vi "Simple_REPL_Comm2.vi"(8 "REPL Name":string="Backpack", 9 "CodeRef":refnum<vi>, 11 "Microprocessor in":T1) -> (3 "Microprocessor out":T1)   [LabVIEW 2016]
uses:
  uPythonX/uPythonX.xctl
  uPythonX/PythonData.ctl
  <vilib>/event_ctls.llb/eventvkey.ctl
  <vilib>/Utility/miscctls.llb/LVPointTypeDef.ctl
panel:
  in  "Help Button":bool
  in  "Find Port":bool
  out "return?":bool
  in  "Board":bool
  out "mouse down?":bool
  in  "Port":string
  out "rows":string
  in  "View":u16(ring) items=["Complete Code"]
  in  "Spaces":bool
  in  "HelpCode":string
  in  "Code":string
  out "Script":string
  in  "Copy":bool
  out "String":string
  in  "Run":bool
  in  "Clear":bool
  in  "Run DIrect":bool
  out "FullCode":string
  out "Origin":T2
  out "Console":string
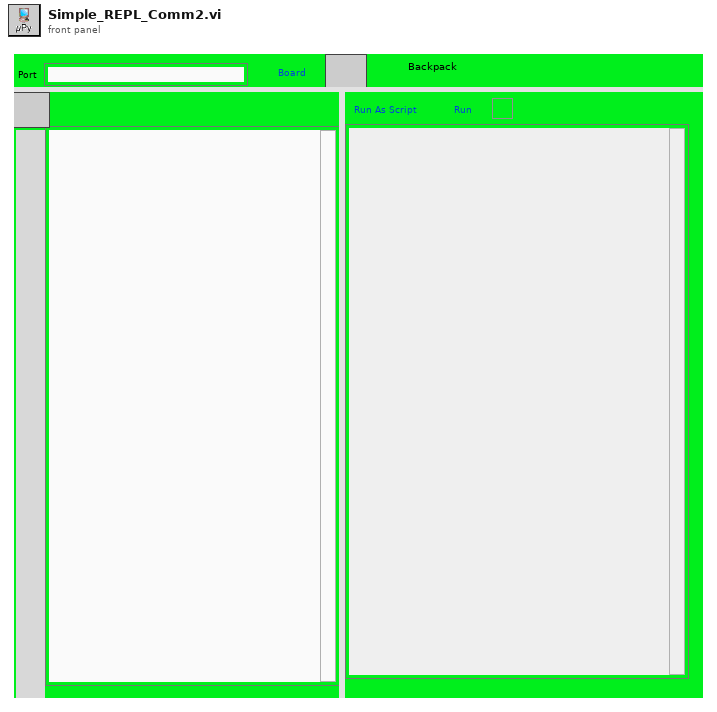
[diagram p1: front panel]
types:
  T1 = cluster{"VISA Refnum in":refnum<visa-resource-name>, "Python Code":string}
  T2 = typedef "LVPointTypeDef.ctl" = cluster{"Horizontal":i16, "Vertical":i16}
  T3 = typedef "uPythonX.xctl/PythonData.ctl" = cluster{"Port":refnum<visa-resource-name>, "All Code":string}
  T4 = typedef "eventvkey.ctl" = enum16{"ASCII", "Enter", "Return", "Shift", "Ctrl", "Alt", "Cmd", "Opt", "Caps", "NumLock", "Clear", "Break", "Up", "Down", "Left", "Right", "Insert", "Delete", "Home", "End", "PageUp", "PageDown", "Escape", "Help", "Pause", "ScrollLock", "F1", "F2", "F3", "F4", "F5", "F6", "F7", "F8", "F9", "F10", "F11", "F12", "F13", "F14", "F15", "F16", "F17", "F18", "F19", "F20", "F21", "F22", "F23", "F24", "Play", "VolumeUp", "VolumeDown", "Mute", "Two Byte Char"}
  T5 = cluster{"Shift":bool, "Ctrl":bool, "Alt":bool, "Cmd":bool, "Opt":bool}
  T6 = cluster{"Char":i16, "VKey":T4, "ScanCode":i16, "Mods":cluster{"Num Pad":bool, "Menu Key":bool}, "PlatMods":cluster{"Shift":bool, "Ctrl":bool, "Alt":bool, "Cmd":bool, "Opt":bool}, "FocusObj":refnum<vi>}
  T7 = enum16{"Left Button", "Center Button", "Right Button", "Window Close"}
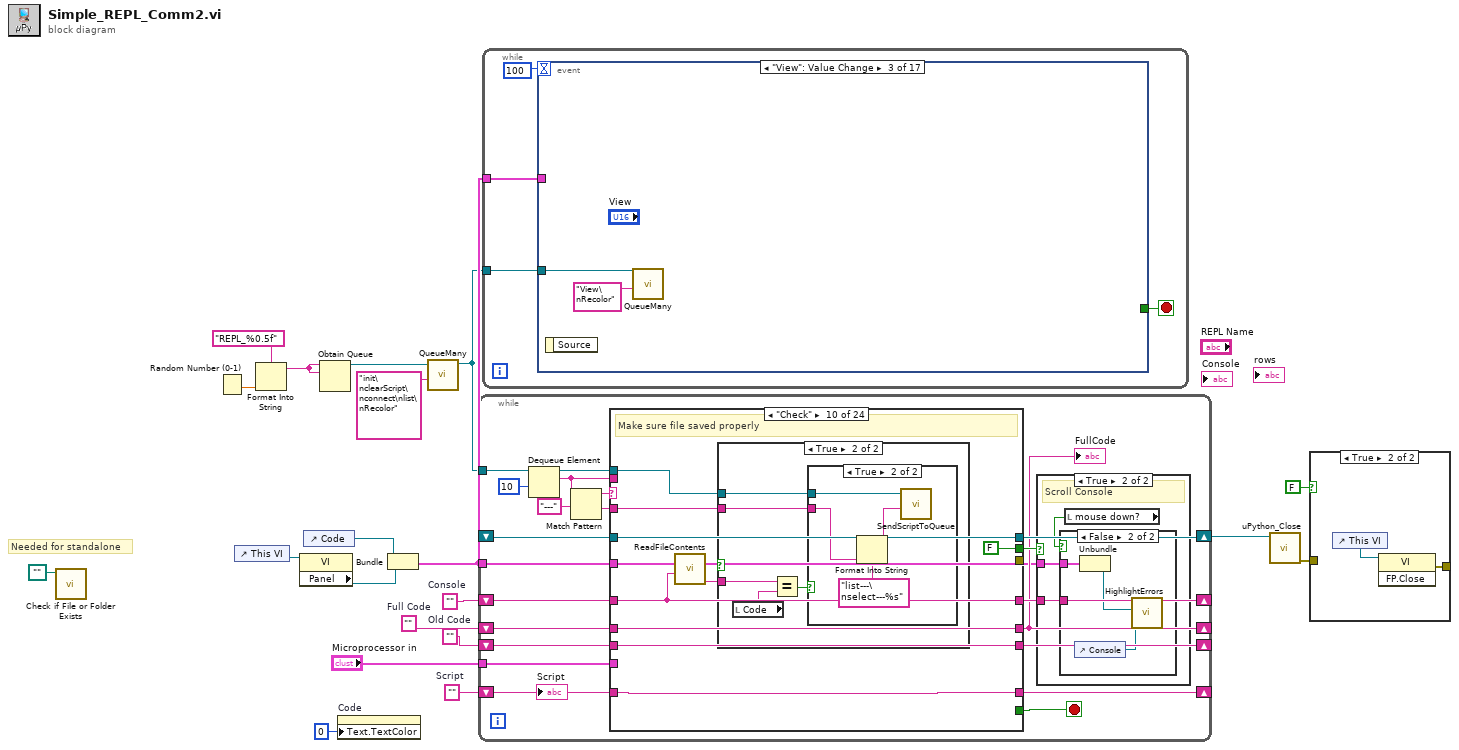
[diagram p0: block diagram]
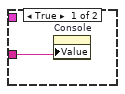
[diagram p4: hidden frame]
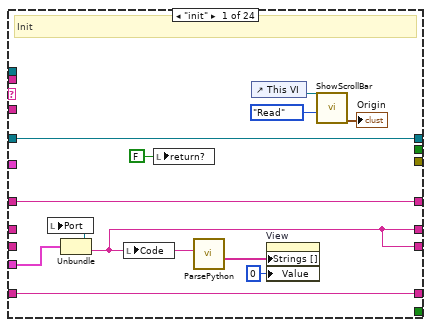
[diagram p5: hidden frame]
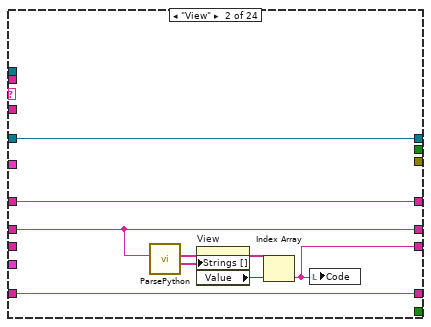
[diagram p6: hidden frame]
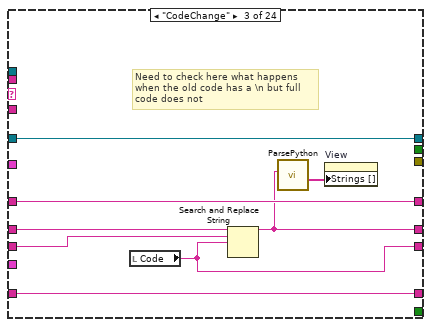
[diagram p7: hidden frame]
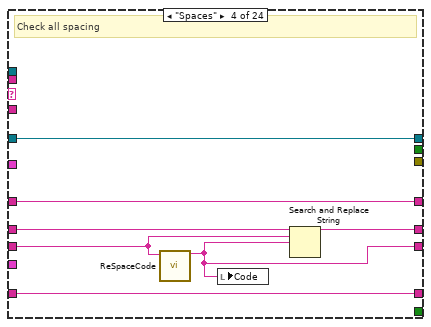
[diagram p8: hidden frame]
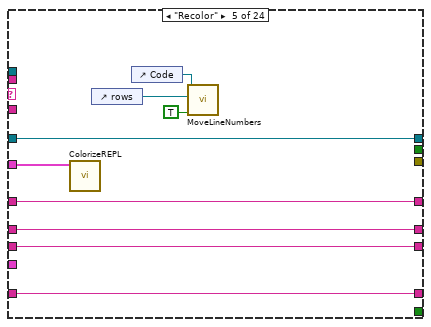
[diagram p9: hidden frame]
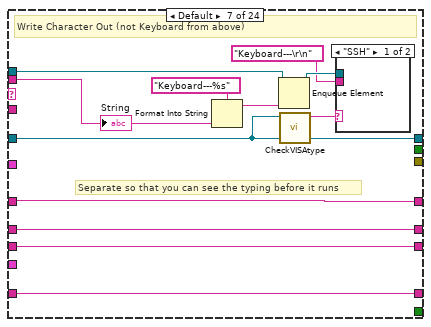
[diagram p11: hidden frame]
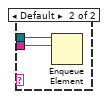
[diagram p12: hidden frame]
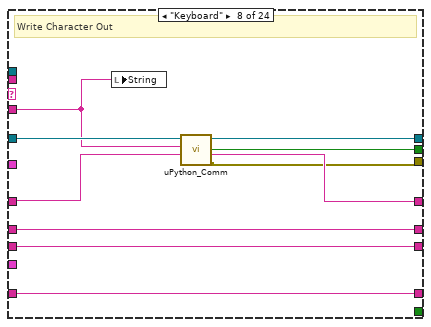
[diagram p13: hidden frame]
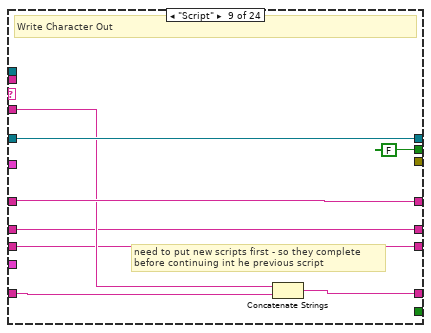
[diagram p14: hidden frame]
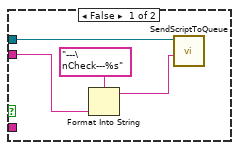
[diagram p15: hidden frame]
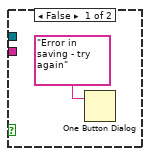
[diagram p16: hidden frame]
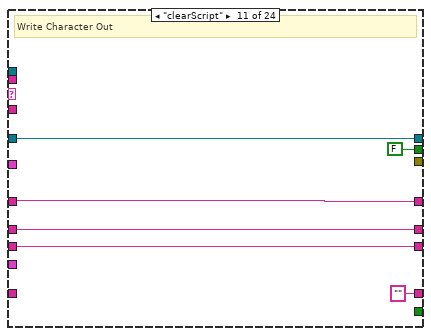
[diagram p17: hidden frame]
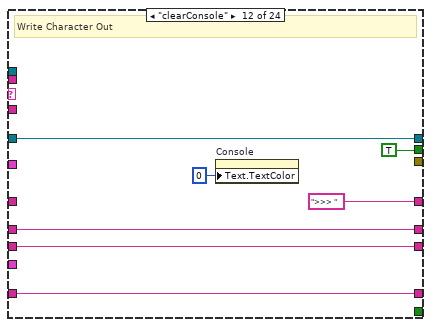
[diagram p18: hidden frame]
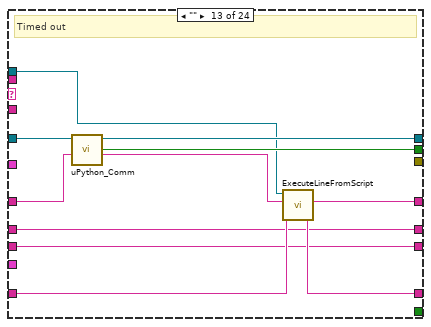
[diagram p19: hidden frame]
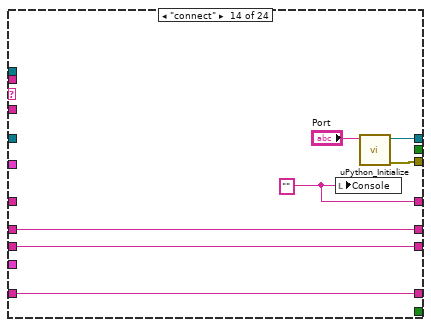
[diagram p20: hidden frame]
diagram:
  w6 = ""  # Old Code
  w7 = ""  # Full Code
  w15 = ""  # Script
  w16 = ""  # Console
  # "Needed for standalone"
  n1 = call <vilib>:"Check if File or Folder Exists.vi"("path"=path "") -> ()  [unwired: 8 in, 3 out]
  n2 = Random Number (0-1)() -> (number: 0 to 1=w10:dbl)
  n3 = control-ref of="This VI"() -> (w5:refnum<vi>)
  n4 = Format Into String(format string="REPL_%0.5f" ("name (unnamed)"), w10) -> (resulting string=w9:string)  [unwired: 2 in, 1 out]
  n5 = property class="VI"(reference=w5) -> ("Panel"=w3:refnum<vi>)  [unwired: 1 in, 2 out]
  n6 = control-ref of="Code"() -> (w4:refnum<vi>)
  n7 = Obtain Queue(name (unnamed)=w9, element data type=w9) -> (queue out=w19:refnum<queue>)  [unwired: 3 in, 2 out]
  n8 = property on="Code" class="Str"("Text.TextColor"=u32 0 ("Text.Text Colors:Text Color")) -> ()  [unwired: 2 in, 2 out]
  n9 = Bundle("Code"=w4, "Panel"=w3) -> (w20:cluster{"Code":refnum<vi>, "Panel":refnum<vi>})  [unwired: 1 in]
  n10 = call "QueueMany.vi"("Playlist"="init\nclearScript\nconnect\nlist\nRecolor" ("element"), "Queue in"=w19) -> ("Queue out"=w18:refnum<queue>)  [unwired: 9 in]
  n11 = while {
    tunnel: w18 -> [w41]
    shift-right: [w31] -> w17
    shift-left: _ -> [w39]
    shift-right: [w30] -> _
    shift-left: w16 -> [w32]
    shift-right: [w28] -> _
    shift-left: w15 -> [w27]
    tunnel: "Microprocessor in" -> [w26]
    shift-right: [w24] -> _
    shift-left: w7 -> [w25]
    shift-right: [w23] -> _
    shift-left: w6 -> [w22]
    tunnel: w20 -> [w21]
    stop <- w40 stop-if-true
    n12 = Dequeue Element(queue=w41, timeout in ms (-1)=10) -> (queue out=w37:refnum<queue>, element=w33:string)  [unwired: 1 in, 2 out]
    n13 = Match Pattern(string=w33, regular expression="---") -> (before substring=w35:string, after substring=w34:string)  [unwired: 1 in, 2 out]
    n14 = case shown="\"Check\"" w35 {
      tunnel: [_ _ _ _ _ _ _ _ _ _ _ _ _ _ _ _ _ _ _ _ _ _ _ TRUE] -> w40
      tunnel: w39 -> [w61 w69 w77 w84 w93 w98 w100 w121 w130 w140 w160 w167 w175 _ w186 w200 w208 w212 w240 w253 w264 w270 w276 w289]
      tunnel: w37 -> [_ _ _ _ _ _ w103 _ _ w136 _ _ w168 _ w190 w197 _ _ _ _ _ _ _ _]
      tunnel: w34 -> [_ _ _ _ _ _ _ w116 w125 w133 _ _ _ _ _ _ _ _ _ _ _ _ _ _]
      tunnel: w33 -> [_ _ _ _ _ _ w105 _ _ _ _ _ _ _ _ _ _ _ _ _ _ _ _ _]
      tunnel: [w61 w69 w77 w84 w93 w98 w100 w119 w130 w140 w160 w167 w172 w184 w186 w200 w208 w220 w244 w250 w264 w270 w276 w289] -> w31
      tunnel: w32 -> [w60 w68 w76 w83 w92 w97 w109 w120 w129 w135 w159 _ w174 _ w189 w199 w207 w215 w241 w254 w266 w272 w278 w290]
      tunnel: [w60 w68 w76 w83 w92 w97 w109 w118 w129 w135 w159 ">>> " ("Console") w173 w182 w189 w199 w207 w218 w228 w248 w266 w272 w278 w290] -> w30
      tunnel: [_ _ _ _ _ _ _ w113 _ _ _ _ _ w183 _ _ _ w217 w243 w249 _ _ _ _] -> _
      tunnel: [_ _ _ _ _ _ _ w117 FALSE ("Update?") FALSE ("Update?") FALSE ("Update?") TRUE ("Update?") w171 _ TRUE ("Update?") _ _ TRUE ("Update?") TRUE ("Update?") TRUE ("Update?") _ _ _ _] -> w29
      tunnel: [w59 w67 w75 w82 w90 w96 w110 w122 w127 w138 "" ("Script") w165 w177 w181 w191 w201 w204 w226 w246 w256 w265 w271 w277 w287] -> w28
      tunnel: w27 -> [w59 w67 w75 w82 w90 w96 w110 w122 w126 w138 _ w165 w176 w181 w191 w201 w204 w226 w246 w256 w265 w271 w277 w287]
      tunnel: w26 -> [w58 _ _ _ _ _ _ _ _ _ _ _ _ _ _ _ _ _ _ _ _ _ _ w286]
      tunnel: [w51 w65 w70 w78 w89 w95 w102 w115 w124 w132 w156 w163 w170 w180 w188 w196 w206 w211 w239 w252 w258 w268 w275 w282] -> w24
      tunnel: w25 -> [_ w65 w74 w81 w89 w95 w102 w115 w124 w132 w156 w163 w170 w180 w188 _ w206 w211 w239 w252 w258 w268 w275 w282]
      tunnel: [w51 w62 w72 w79 w91 w94 w101 w114 w123 w131 w155 w162 w169 w179 w187 w196 w205 w210 w238 w251 w257 w267 w274 w281] -> w23
      tunnel: w22 -> [_ _ w73 w80 w91 w94 w101 w114 w123 w131 w155 w162 w169 w179 w187 _ w205 w210 w238 w251 w257 w267 w274 w281]
      tunnel: w21 -> [_ _ _ _ w88 _ _ _ _ _ _ _ _ _ _ _ _ _ _ _ _ _ _ _]
      frame "init" {
        # "Init"
        n15 = Unbundle(w58) -> ("VISA Refnum in"=w54:refnum<visa-resource-name>, "Python Code"=w51:string)
        n16 = local write "Port"(w54) -> ()
        n17 = local write "Code"(w51) -> ()
        n18 = local write "return?"(FALSE ("return?")) -> ()
        n19 = call "ParsePython.vi"("String"=w51) -> ("functions"=w53:string[])  [unwired: 8 in, 2 out]
        n20 = control-ref of="This VI"() -> (w57:refnum<vi>)
        n21 = property on="View" class="Ring (strict)"("Strings []"=w53, "Value"=0 ("timeout in ms (-1)")) -> ()  [unwired: 2 in, 2 out]
        n22 = call "ShowScrollBar.vi"("Task"=enum16{"Read", "Open", "Close", "Reset"}."Read", "VI in"=w57) -> ("Origin"=→"Origin":T2)  [unwired: 9 in]
      }
      frame "View" {
        n23 = call "ParsePython.vi"("String"=w65) -> ("functions"=w64:string[], "Subs"=w63:string[])  [unwired: 8 in, 1 out]
        n24 = property on="View" class="Ring (strict)"("Strings []"=w64) -> ("Value"=w66:u16)  [unwired: 2 in, 2 out]
        n25 = Index Array(array=w63, index=w66) -> (element=w62:string)
        n26 = local write "Code"(w62) -> ()
      }
      frame "CodeChange" {
        # "Need to check here what happens\nwhen the old code has a \\n but full\ncode does not"
        n27 = local read "Code"() -> (w72:string)
        n28 = Search and Replace String(input string=w74, search string=w73, replace string=w72) -> (result string=w70:string)  [unwired: 5 in, 3 out]
        n29 = call "ParsePython.vi"("String"=w70) -> ("functions"=w71:string[])  [unwired: 8 in, 2 out]
        n30 = property on="View" class="Ring (strict)"("Strings []"=w71) -> ()  [unwired: 2 in, 2 out]
      }
      frame "Spaces" {
        # "Check all spacing"
        n31 = call "ReSpaceCode.vi"("Code"=w80) -> ("String"=w79:string)  [unwired: 10 in]
        n32 = local write "Code"(w79) -> ()
        n33 = Search and Replace String(input string=w81, search string=w80, replace string=w79) -> (result string=w78:string)  [unwired: 5 in, 3 out]
      }
      frame "Recolor" {
        n34 = call "ColorizeREPL.vi"("refs"=w88) -> ()  [unwired: 9 in, 1 out]
        n35 = control-ref of="rows"() -> (w86:refnum<vi>)
        n36 = control-ref of="Code"() -> (w87:refnum<vi>)
        n37 = call "MoveLineNumbers.vi"("Force?"=TRUE, "rows"=w86, "Code"=w87) -> ()  [unwired: 9 in]
      }
      frame "scroll" {
        # "reset row numbers"
      }
      frame Default {
        # "Separate so that you can see the typing before it runs"
        # "Write Character Out (not Keyboard from above)"
        n38 = Format Into String(format string="Keyboard---%s", w105) -> (resulting string=w107:string)  [unwired: 2 in, 1 out]
        n39 = Enqueue Element(queue=w103, element=w107) -> (queue out=w106:refnum<queue>)  [unwired: 2 in, 2 out]
        n40 = call "CheckVISAtype.vi"("VISA Refnum in"=w100) -> ("data string"=w99:string)  [unwired: 8 in, 2 out]
        n41 = case shown="\"SSH\"" w99 {
          tunnel: w106 -> [_ w112]
          tunnel: "Keyboard---\r\n" ("regular expression") -> [_ w111]
          frame "SSH" {
          }
          frame Default {
            n42 = Enqueue Element(queue=w112, element=w111) -> ()  [unwired: 2 in, 3 out]
          }
        }
        "String" <- w105
      }
      frame "Keyboard" {
        # "Write Character Out"
        n43 = local write "String"(w116) -> ()
        n44 = call "uPython_Comm.vi"("Console In"=w120, "Script"=w116, "VISA Refnum in"=w121) -> ("error out"=w113:errorcluster, "Console Out"=w118:string, "VISA out"=w119:refnum<visa-resource-name>, "Update?"=w117:bool)  [unwired: 4 in, 1 out]
      }
      frame "Script" {
        # "need to put new scripts first - so they complete\nbefore continuing int he previous script"
        # "Write Character Out"
        n45 = Concatenate Strings(w125, w126) -> (w127:string)
      }
      frame "Check" {
        # "Make sure file saved properly"
        n46 = call "ReadFileContents.vi"("Console"=w135) -> ("File Contents"=w134:string, "Success?"=w137:bool)  [unwired: 9 in]
        n47 = case shown="True" w137 {
          tunnel: w136 -> [w144 w145]
          tunnel: w134 -> [_ w148]
          tunnel: w133 -> [w142 w147]
          frame False {
            n48 = Format Into String(format string="---\nCheck---%s" ("String"), w142) -> (resulting string=w141:string)  [unwired: 2 in, 1 out]
            n49 = call "SendScriptToQueue.vi"("String"=w141, "Queue in"=w144) -> ()  [unwired: 10 in]
          }
          frame True {
            n50 = local read "Code"() -> (w149:string)
            n51 = Equal?(x=w148, y=w149) -> (x = y?=w146:bool)
            n52 = case shown="True" w146 {
              tunnel: w147 -> [_ w153]
              tunnel: w145 -> [_ w152]
              frame False {
                n53 = One Button Dialog(message="Error in saving - try again" ("Code")) -> ()  [unwired: 1 in, 1 out]
              }
              frame True {
                n54 = Format Into String(format string="list---\nselect---%s" ("element"), w153) -> (resulting string=w151:string)  [unwired: 2 in, 1 out]
                n55 = call "SendScriptToQueue.vi"("String"=w151, "Queue in"=w152) -> ()  [unwired: 10 in]
              }
            }
          }
        }
      }
      frame "clearScript" {
        # "Write Character Out"
      }
      frame "clearConsole" {
        # "Write Character Out"
        n56 = property on="Console" class="Str"("Text.TextColor"=u32 0 ("Text.Text Colors:Text Color")) -> ()  [unwired: 2 in, 2 out]
      }
      frame "" {
        # "Timed out"
        n57 = call "uPython_Comm.vi"("Console In"=w174, "VISA Refnum in"=w175) -> ("Console Out"=w173:string, "VISA out"=w172:refnum<visa-resource-name>, "Update?"=w171:bool)  [unwired: 5 in, 2 out]
        n58 = call "ExecuteLineFromScript.vi"("Script in"=w176, "Console"=w173, "Queue in"=w168) -> ("Script out"=w177:string)  [unwired: 8 in]
      }
      frame "connect" {
        w182 = "" ("element")
        n59 = local write "Console"(w182) -> ()
        n60 = call "uPython_Initialize.vi"("VISA Refnum in"="Port") -> ("error out"=w183:errorcluster, "VISA Refnum out"=w184:refnum<visa-resource-name>)  [unwired: 9 in]
      }
      frame "list" {
        # "get file listing"
        n61 = call "CheckVISAtype.vi"("VISA Refnum in"=w186) -> ("data string"=w185:string)  [unwired: 8 in, 2 out]
        n62 = case shown="Default" w185 {
          tunnel: w190 -> [w194 _]
          frame Default {
            n63 = call "SendScriptToQueue.vi"("String"="import os\nos.listdir()\n\nlisting---" ("element"), "Queue in"=w194) -> ()  [unwired: 10 in]
          }
          frame "" {
          }
        }
      }
      frame "read" {
        n64 = call "ReadFileContents.vi"("Console"=w199) -> ("File Contents"=w196:string, "Success?"=w198:bool)  [unwired: 9 in]
        n65 = local write "Code"(w196) -> ()
        n66 = case shown="False" w198 {
          tunnel: w197 -> [w203 _]
          frame False {
            n67 = call "SendScriptToQueue.vi"("String"="---\nread---", "Queue in"=w203) -> ()  [unwired: 10 in]
          }
          frame True {
          }
        }
        n68 = property on="View" class="Ring (strict)"("Val(Sgnl)"=0 ("timeout in ms (-1)")) -> ()  [unwired: 2 in, 2 out]
      }
      frame "ListDialog" {
        n69 = call "ReadFilesOnMP.vi"("VISA"=w208) -> ()  [unwired: 11 in]
      }
      frame "run" {
        w216 = "\u0003"  # Ctrl C
        w223 = "\u0004"  # Ctrl D
        # "run on main.py"
        n70 = call "uPython_Comm.vi"("Console In"=w215, "Script"=w216, "VISA Refnum in"=w212) -> ("error out"=w214:errorcluster, "VISA out"=w213:refnum<visa-resource-name>)  [unwired: 4 in, 3 out]
        n71 = local read "Code"() -> (w219:string)
        n72 = call "SavePyFile.vi"("Name"="main.py", "error in"=w214, "Python Code"=w219, "VISA in"=w213) -> ("error out"=w224:errorcluster, "Reply"=w222:string, "VISA out"=w225:refnum<visa-resource-name>)  [unwired: 5 in]
        n73 = call "uPython_Comm.vi"("error in (no error)"=w224, "Console In"=w222, "Script"=w223, "VISA Refnum in"=w225) -> ("error out"=w217:errorcluster, "Console Out"=w218:string, "VISA out"=w220:refnum<visa-resource-name>)  [unwired: 3 in, 2 out]
      }
      frame "runRaw" {
        w242 = "\u0003\u0003\u0001"  # Ctrl C,C,A
        w245 = "\u0004"  # Ctrl D
        # "run on main.py"
        n74 = call "uPython_Comm.vi"("Console In"=w241, "Script"=w242, "VISA Refnum in"=w240) -> ("error out"=w236:errorcluster, "Console Out"=w232:string, "VISA out"=w237:refnum<visa-resource-name>)  [unwired: 4 in, 2 out]
        n75 = local read "Code"() -> (w233:string)
        n76 = call "uPython_Comm.vi"("error in (no error)"=w236, "Console In"=w232, "Script"=w233, "VISA Refnum in"=w237) -> ("error out"=w235:errorcluster, "Console Out"=w231:string, "VISA out"=w234:refnum<visa-resource-name>)  [unwired: 3 in, 2 out]
        n77 = call "uPython_Comm.vi"("error in (no error)"=w235, "Console In"=w231, "Script"=w245, "VISA Refnum in"=w234) -> ("error out"=w243:errorcluster, "Console Out"=w229:string, "VISA out"=w244:refnum<visa-resource-name>)  [unwired: 3 in, 2 out]
        n78 = Concatenate Strings(w229, "\r\n" ("Script")) -> (w228:string)
      }
      frame "leaveRaw" {
        w255 = "\r\u0002"  # \r Ctrl B
        # "run on main.py"
        n79 = call "uPython_Comm.vi"("Console In"=w254, "Script"=w255, "VISA Refnum in"=w253) -> ("error out"=w249:errorcluster, "Console Out"=w248:string, "VISA out"=w250:refnum<visa-resource-name>)  [unwired: 4 in, 2 out]
      }
      frame "help" {
        n80 = local read "Code"() -> (w259:string)
        n81 = Bundle(cluster=T3 {"Port"="", "All Code"="Hi"} ("Data In"), "Port"=w264, "All Code"=w259) -> (w263:T3)
        n82 = control-ref of="HelpCode"() -> (w261:refnum<vi>)
        n83 = call "OpenHelp.vi"("Code Ref"=w261, "Data In"=w263, "Dialog"=enum16{"REPL", "Help"}."Help") -> ()  [unwired: 9 in]
      }
      frame "update" {
        n84 = property class="Str"(reference="CodeRef", "Val(Sgnl)"=w268) -> ()  [unwired: 1 in, 2 out]
      }
      frame "findPort" {
        n85 = call "GatheringSerialPortNames.vi"() -> ("name"=w273:string)  [unwired: 11 in]
        n86 = property on="Port" class="Str"("Val(Sgnl)"=w273) -> ()  [unwired: 2 in, 2 out]
      }
      frame "done" {
        n87 = property on="Code" class="Str"("Value"="" ("Code"), "Text.TextColor"=u32 0 ("Text.Text Colors:Text Color")) -> ()  [unwired: 2 in, 2 out]
        n88 = Bundle(cluster=w286, "VISA Refnum in"=w289, "Python Code"=w282) -> (→"Microprocessor out":T1)
        n89 = control-ref of="This VI"() -> (w284:refnum<vi>)
        n90 = local read "Origin"() -> (w285:T2)
        n91 = call "ShowScrollBar.vi"("Origin in"=w285, "Task"=enum16{"Read", "Open", "Close", "Reset"}."Reset", "VI in"=w284) -> ()  [unwired: 8 in, 1 out]
      }
    }
    "FullCode" <- w24
    n92 = case shown="True" w29 {
      tunnel: w30 -> [_ w44]
      tunnel: w21 -> [_ w42]
      frame False {
      }
      frame True {
        # "Scroll Console"
        n93 = local read "mouse down?"() -> (w43:bool)
        n94 = case shown="False" w43 {
          tunnel: w44 -> [w45 w49]
          tunnel: w42 -> [_ w47]
          frame True {
            n95 = property on="Console" class="Str"("Value"=w45) -> ()  [unwired: 2 in, 2 out]
          }
          frame False {
            n96 = control-ref of="Console"() -> (w48:refnum<vi>)
            n97 = Unbundle(w47) -> ("Panel"=w46:refnum<vi>)  [unwired: 1 out]
            n98 = call "HighlightErrors.vi"("String"=w49, "Front Panel"=w46, "Console"=w48) -> ()  [unwired: 9 in]
          }
        }
      }
    }
    "Script" <- w27
  }
  n99 = while {
    tunnel: w18 -> [w295]
    tunnel: w20 -> [w292]
    stop <- w294 stop-if-true
    n100 = event shown="[2] \"View\": Value Change" {
      selector: _ -> [_ _ _ _ _ _ _ _ _ _ _ _ _ _ _ _ _]
      dyn-events: _ -> [_ _ _ _ _ _ _ _ _ _ _ _ _ _ _ _ _]
      timeout: 100 -> [_ _ _ _ _ _ _ _ _ _ _ _ _ _ _ _ _]
      tunnel: w295 -> [_ w301 w304 w306 w312 w330 _ _ w340 w353 w355 w357 w358 w360 w362 _ w365]
      tunnel: [_ _ _ _ _ _ _ _ w333 _ _ _ _ _ _ _ _] -> w294
      tunnel: w292 -> [_ w300 _ _ _ _ _ _ _ _ _ _ _ _ _ _ _]
      event Timeout {
        n101 = event-data() -> ()  [unwired: 1 in, 3 out]
        n102 = control-ref of="Code"() -> (w297:refnum<vi>)
        n103 = control-ref of="rows"() -> (w298:refnum<vi>)
        n104 = call "MoveLineNumbers.vi"("Force?"=TRUE, "rows"=w298, "Code"=w297) -> ()  [unwired: 9 in]
      }
      event "Code": Value Change {
        # "Need to have these here or you can get screwy stuff happening"
        n105 = event-data() -> ()  [unwired: 1 in, 2 out]
        n106 = local read "return?"() -> (w299:bool)
        n107 = call "ColorizeREPL.vi"("refs"=w300, "Add Spaces?"=w299) -> ()  [unwired: 8 in, 1 out]
        n108 = call "QueueMany.vi"("Playlist"="CodeChange" ("element"), "Queue in"=w301) -> ()  [unwired: 9 in, 1 out]
      }
      event "View": Value Change {
        n109 = event-data() -> ()  [unwired: 1 in, 1 out]
        n110 = call "QueueMany.vi"("Playlist"="View\nRecolor" ("element"), "Queue in"=w304) -> ()  [unwired: 9 in, 1 out]
      }
      event "Spaces": Value Change {
        n111 = event-data() -> ()  [unwired: 1 in, 1 out]
        n112 = call "QueueMany.vi"("Playlist"="Spaces\nRecolor" ("element"), "Queue in"=w306) -> ()  [unwired: 9 in, 1 out]
      }
      event Key Down {
        n113 = event-data() -> ("Char"=w316:i16, "VKey"=w307:T4, "ScanCode"=w315:i16, "Mods"=w314:cluster{"Num Pad":bool, "Menu Key":bool}, "PlatMods"=w313:T5, "FocusObj"=w309:refnum<vi>)  [unwired: 1 in]
        n114 = Bundle("Char"=w316, "VKey"=w307, "ScanCode"=w315, "Mods"=w314, "PlatMods"=w313, "FocusObj"=w309) -> (w317:T6)  [unwired: 1 in]
        n115 = control-ref of="Code"() -> (w310:refnum<vi>)
        n116 = Not Equal?(x=w310, y=w309) -> (x != y?=w311:bool)
        n117 = case shown="False" w311 {
          tunnel: w317 -> [_ w324]
          tunnel: w312 -> [_ w322]
          tunnel: w307 -> [w319 _]
          tunnel: [w318 _] -> w308
          frame False {
            n118 = Equal?(x=eventvkey."Return" ("VKey"), y=w319) -> (x = y?=w318:bool)
          }
          frame True {
            n119 = call "TranslateTyping.vi"("Cluster"=w324) -> ("Script?"=w321:bool, "string"=w323:string)  [unwired: 8 in, 1 out]
            n120 = case shown="True" w321 {
              tunnel: w323 -> [w325 w328]
              tunnel: w322 -> [w326 w327]
              frame False {
                n121 = call "QueueMany.vi"("Playlist"=w325, "Queue in"=w326) -> ()  [unwired: 9 in, 1 out]
              }
              frame True {
                n122 = call "SendScriptToQueue.vi"("String"=w328, "Queue in"=w327) -> ()  [unwired: 10 in]
              }
            }
          }
        }
        "return?" <- w308
      }
      event "Copy": Value Change {
        n123 = event-data() -> ()  [unwired: 1 in, 1 out]
        n124 = call "QueueMany.vi"("Playlist"="update" ("element"), "Queue in"=w330) -> ()  [unwired: 9 in, 1 out]
      }
      event Mouse Down {
        n125 = event-data() -> ()  [unwired: 1 in, 8 out]
        "mouse down?" <- TRUE ("mouse down?")
      }
      event Mouse Leave; Mouse Up {
        n126 = event-data() -> ()  [unwired: 1 in, 4 out]
        n127 = local write "mouse down?"(FALSE ("mouse down?")) -> ()
      }
      event Panel Close? {
        n128 = event-data() -> ()  [unwired: 1 in, 1 out]
        n129 = local read "Microprocessor in"() -> (w337:T1)
        n130 = local read "Code"() -> (w336:string)
        n131 = Unbundle By Name(w337) -> ("Python Code"=w335:string)
        n132 = Not Equal?(x=w335, y=w336) -> (x != y?=w334:bool)
        n133 = case shown="True" w334 {
          tunnel: ["done" ("element") w345] -> w338
          tunnel: [TRUE ("Discard?") w344] -> w333
          frame False {
          }
          frame True {
            n134 = call "CloseDialog.vi"() -> ("Which Button?"=w343:T7)  [unwired: 11 in]
            n135 = case shown="\"Center Button\"" w343 {
              tunnel: ["update\ndone" ("element") "done" ("element") "" ("element")] -> w345
              tunnel: [TRUE ("Discard?") TRUE ("Discard?") FALSE ("Discard?")] -> w344
              frame "Left Button" {
              }
              frame "Center Button" {
              }
              frame Default {
              }
            }
          }
        }
        n136 = call "QueueMany.vi"("Playlist"=w338, "Queue in"=w340) -> ()  [unwired: 9 in, 1 out]
        n137 = event-data("Discard?"=TRUE) -> ()  [unwired: 1 in, 1 out]
      }
      event "Board": Value Change {
        n138 = event-data() -> ()  [unwired: 1 in, 1 out]
        n139 = call "QueueMany.vi"("Playlist"="ListDialog" ("element"), "Queue in"=w353) -> ()  [unwired: 9 in, 1 out]
      }
      event "Find Port": Value Change {
        n140 = event-data() -> ()  [unwired: 1 in, 1 out]
        n141 = call "QueueMany.vi"("Playlist"="findPort" ("element"), "Queue in"=w355) -> ()  [unwired: 9 in, 1 out]
      }
      event "Run DIrect": Value Change {
        n142 = event-data() -> ()  [unwired: 1 in, 1 out]
        n143 = call "SendScriptToQueue.vi"("String"="Code", "Queue in"=w357) -> ()  [unwired: 10 in]
      }
      event "Run": Value Change {
        n144 = event-data() -> ()  [unwired: 1 in, 1 out]
        n145 = call "QueueMany.vi"("Playlist"="runRaw" ("element"), "Queue in"=w358) -> ()  [unwired: 9 in, 1 out]
      }
      event "Port": Value Change {
        n146 = event-data() -> ()  [unwired: 1 in, 1 out]
        n147 = call "QueueMany.vi"("Playlist"="connect\nlist" ("element"), "Queue in"=w360) -> ()  [unwired: 9 in, 1 out]
      }
      event "Help Button": Value Change {
        n148 = event-data() -> ()  [unwired: 1 in, 1 out]
        n149 = call "QueueMany.vi"("Playlist"="help" ("element"), "Queue in"=w362) -> ()  [unwired: 9 in, 1 out]
      }
      event "HelpCode": Value Change {
        n150 = event-data() -> ()  [unwired: 1 in, 1 out]
        n151 = property on="Code" class="Str"("Val(Sgnl)"="HelpCode") -> ()  [unwired: 2 in, 2 out]
      }
      event "Clear": Value Change {
        n152 = event-data() -> ()  [unwired: 1 in, 2 out]
        n153 = call "QueueMany.vi"("Playlist"="clearConsole" ("element"), "Queue in"=w365) -> ()  [unwired: 9 in, 1 out]
      }
    }
  }
  n154 = call "uPython_Close.vi"("VISA  in"=w17) -> ("error out"=w13:errorcluster)  [unwired: 9 in, 1 out]
  n155 = case shown="True" FALSE {
    tunnel: w13 -> [_ _]
    tunnel: [_ w367] -> _
    frame False {
    }
    frame True {
      n156 = control-ref of="This VI"() -> (w368:refnum<vi>)
      n157 = invoke class="VI" method="FP.Close"(reference=w368) -> (error out=w367:errorcluster)  [unwired: 2 in, 2 out]
    }
  }
